vi "Read Waveform Measurement (Px Statistics).vi"(0 "VISA resource name":refnum<visa-resource-name>, 5 "Parameter (0: P1)":u16(ring) items=["P1", "P2", "P3", "P4", "P5", "P6", "P7", "P8"], 11 "error in (no error)":errorcluster) -> (2 "Min":dbl format="%#_6e", 3 "Max":dbl format="%#_6e", 4 "VISA resource name out":refnum<visa-resource-name>, 6 "Value":dbl format="%#_6e", 8 "Sigma":dbl format="%#_6e", 10 "num":dbl format="%#_6f", 12 "StatusDescription":string, 13 "Mean":dbl format="%#_6e", 14 "enabled?":bool, 15 "error out":errorcluster)   [LabVIEW 2020, in "LeCroy Wave Series.lvlib"]
doc: "This VI reads back all statistics for a parameter previously configured on P1 - P8. P1-P5 are available on most scopes; availability is model dependant.\n\n(The statistics table does not need to be visible on the scope to use this VI)"
uses:
  LeCroy Wave Series.lvlib
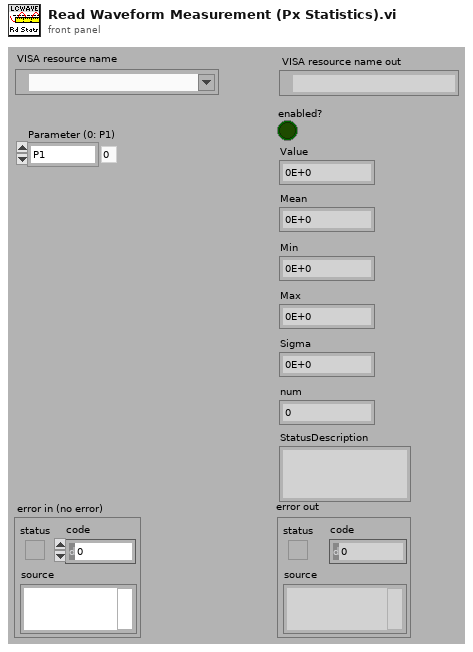
[diagram p1: front panel]
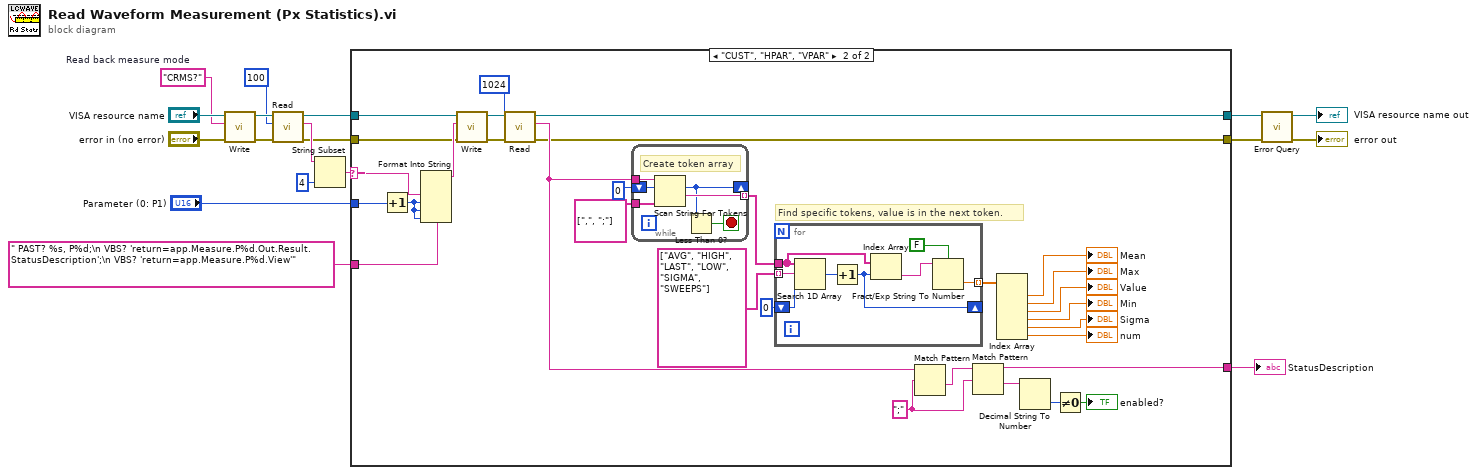
[diagram p0: block diagram]
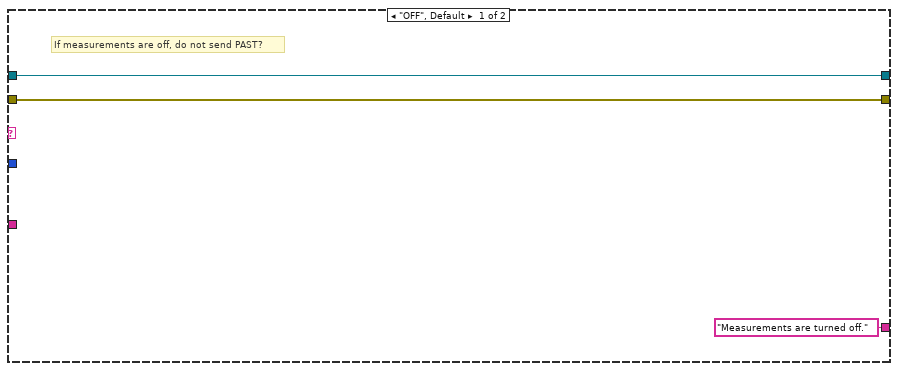
[diagram p2: hidden frame]
diagram:
  w14 = "CRMS?"  # Read back measure mode
  n1 = call "Write.vi"("error in (no error)"="error in (no error)", "Write Buffer"=w14, "VISA resource name"="VISA resource name") -> ("error out"=w13:errorcluster, "VISA resource name out"=w17:refnum<visa-resource-name>)  [unwired: 6 in, 1 out]
  n2 = call "Read.vi"("error in (no error)"=w13, "Byte Count"=u32 100, "VISA resource name"=w17) -> ("error out"=w6:errorcluster, "Read Buffer"=w8:string, "VISA resource name out"=w11:refnum<visa-resource-name>)  [unwired: 5 in, 1 out]
  n3 = String Subset(string=w8, length (rest)=4 ("length (rest)")) -> (substring=w7:string)  [unwired: 1 in]
  n4 = case shown="\"CUST\", \"HPAR\", \"VPAR\"" w7 {
    selector: w7 -> [_ w26]
    tunnel: ["Measurements are turned off." ("Read Buffer") w30] -> w18
    tunnel: w11 -> [w19 w29]
    tunnel: "Parameter (0: P1)" -> [_ w27]
    tunnel: w6 -> [w20 w25]
    tunnel: [w20 w24] -> w3
    tunnel: [w19 w23] -> w2
    tunnel: " PAST? %s, P%d;\n VBS? 'return=app.Measure.P%d.Out.Result.StatusDescription';\n VBS? 'return=app.Measure.P%d.View'" ("format string") -> [_ w22]
    frame "OFF", Default {
      # "If measurements are off, do not send PAST?"
    }
    frame "CUST", "HPAR", "VPAR" {
      w34 = ";" ("regular expression")
      # "Find specific tokens, value is in the next token."
      n5 = Increment(x=w27) -> (x+1=w28:u16)
      n6 = Format Into String(format string=w22, w26, w28, w28, w28) -> (resulting string=w50:string)  [unwired: 2 in, 1 out]
      n7 = call "Write.vi"("error in (no error)"=w25, "Write Buffer"=w50, "VISA resource name"=w29) -> ("error out"=w51:errorcluster, "VISA resource name out"=w52:refnum<visa-resource-name>)  [unwired: 6 in, 1 out]
      n8 = call "Read.vi"("error in (no error)"=w51, "Byte Count"=u32 1024, "VISA resource name"=w52) -> ("error out"=w24:errorcluster, "Read Buffer"=w36:string, "VISA resource name out"=w23:refnum<visa-resource-name>)  [unwired: 5 in, 1 out]
      n9 = while {
        tunnel: w36 -> [w66]
        tunnel: string[] [",", ";"] ("delimiters (\\s,\\t,\\r,\\n)") -> [w65]
        shift-right: [w61] -> _
        shift-left: 0 ("offset past token") -> [w64]
        tunnel: [w63] -> w45 mode=indexing
        stop <- w62 stop-if-true
        # "Create token array"
        n10 = Scan String For Tokens(6:w65, 8:w64, 9:w66) -> (1:w63:string, 2:w61:i32)  [unwired: 3 in, 2 out]
        n11 = Less Than 0?(x=w61) -> (x < 0?=w62:bool)
      }
      n12 = for {
        tunnel: w45 -> [w56]
        tunnel: string[] ["AVG", "HIGH", "LAST", "LOW", "SIGMA", "SWEEPS"] -> [w60] mode=indexing
        shift-right: [w57] -> _
        shift-left: 0 -> [w58]
        tunnel: [w53] -> w43 mode=indexing
        n13 = Search 1D Array(1D array=w56, element=w60, start index (0)=w58) -> (index of element=w59:i32)
        n14 = Increment(x=w59) -> (x+1=w57:i32)
        n15 = Index Array(array=w56, index=w57) -> (element=w55:string)
        n16 = Fract/Exp String To Number(use system decimal point (T)=FALSE, string=w55) -> (number=w53:dbl)  [unwired: 2 in, 1 out]
      }
      n17 = Match Pattern(string=w36, regular expression=w34) -> (after substring=w35:string)  [unwired: 1 in, 3 out]
      n18 = Match Pattern(string=w35, regular expression=w34) -> (before substring=w30:string, after substring=w33:string)  [unwired: 1 in, 2 out]
      n19 = Index Array(array=w43) -> (element #1=→"Mean":dbl, element #2=→"Max":dbl, element #3=→"Value":dbl, element #4=→"Min":dbl, element #5=→"Sigma":dbl, element #6=→"num":dbl)  [unwired: 6 in]
      n20 = Decimal String To Number(string=w33) -> (number=w32:i32)  [unwired: 2 in, 1 out]
      n21 = Not Equal To 0?(x=w32) -> (x != 0?=→"enabled?":bool)
    }
  }
  "StatusDescription" <- w18
  n22 = call "Error Query.vi"("error in (no error)"=w3, "VISA resource name"=w2) -> ("error out"=→"error out":errorcluster, "VISA resource name out"=→"VISA resource name out":refnum<visa-resource-name>)  [unwired: 6 in, 2 out]
